vi "Set Unit ID.vi"(8 "error in (no error)":errorcluster, 10 "unit ID":u8, 11 "Modbus master in":refnum<class "Modbus Master.lvclass">) -> (0 "error out":errorcluster, 3 "Modbus master out":refnum<class "Modbus Master.lvclass">)   [LabVIEW 2018, in "Modbus Master.lvclass"]
doc: "Sets the identification of a serial Modbus slave. When you wire a Modbus master instance to the <b>Modbus master in</b> input and specify a value for the <b>unit ID</b> input, this Modbus master instance can communicate with the Modbus slave with the specified unit ID. This VI ignores requests from TCP Modbus master instances."
uses:
  Modbus Master.lvclass
  C:/Program Files (x86)/National Instruments/LabVIEW 2018/vi.lib/Modbus/subvis/Modbus API/Modbus API.lvclass
  Modbus API.lvclass/Modbus API.ctl
  Transmission Data Unit.lvclass/Transmission Data Unit.ctl
  Write Unit ID.vi
  Read Transmission Data Unit.vi
  Write Transmission Data Unit.vi
  Transmission Data Unit.lvclass
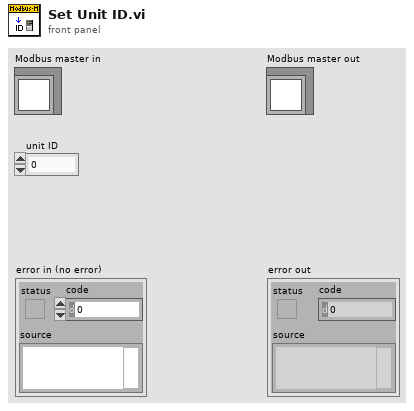
[diagram p1: front panel]
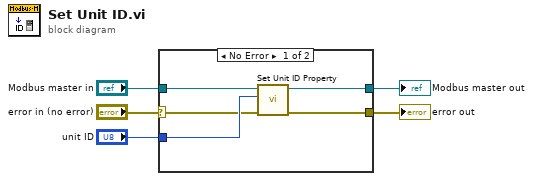
[diagram p0: block diagram]
diagram:
  n1 = case shown="No Error" "error in (no error)" {
    selector: "error in (no error)" -> [w6 w11]
    tunnel: "unit ID" -> [w10 _]
    tunnel: "Modbus master in" -> [w9 w12]
    tunnel: [w8 w12] -> w3
    tunnel: [w7 w11] -> w2
    frame No Error {
      n2 = call "Set Unit ID Property.vi"("error in (no error)"=w6, "unit ID"=w10, "Modbus master in"=w9) -> ("error out"=w7:errorcluster, "Modbus master out"=w8:refnum<class "Modbus Master.lvclass">)  [unwired: 7 in]
    }
    frame Error {
    }
  }
  "error out" <- w2
  "Modbus master out" <- w3
